vi "TimeInterpRotation2d_GetSample.vi"(9 "TimeStamp":dbl, 11 "TimeInterpRotation":T1 {"RotationValues"."SIN" format="%13.4f"; "RotationValues"."COS" format="%13.4f"; "RotationValues"."VALUE" format="%13.4f"}) -> (1 "IsPresent":bool, 3 "OutputRotation":T2={"VALUE"=0.0, "COS"=1.0, "SIN"=0.0} {"SIN" format="%13.4f"; "COS" format="%13.4f"; "VALUE" format="%13.4f"})   [LabVIEW 2019, in "Trajectory_Library.lvlib"]
doc: "Sample the buffer at the given time.\n\nInputs:\n - TimeInterpRotation2d -- Input data cluster\n - TimeStamp -- Time at which to sample (seconds)\n\nOutputs\n - OutputRotation -- Sampled Rotation2d. This is an exact value if there is a sample in the buffer at this time. Otherwise the value is interpolated. \n - IsPresent -- Returns TRUE if the buffer contains data as far back as TimeStamp."
uses:
  Trajectory_Library.lvlib
  <vilib>/gmath/NI_Gmath.lvlib
  ROTATION2D.ctl
  TypeDef/TIME_INTERPOLATABLE_ROTATION2D.ctl
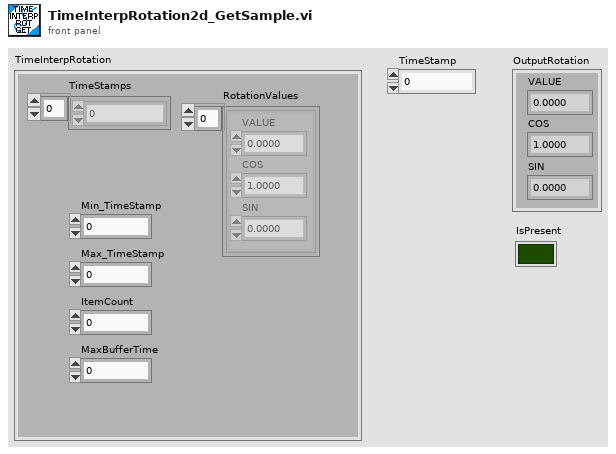
[diagram p1: front panel]
types:
  T1 = typedef "Trajectory_Library.lvlib/TIME_INTERPOLATABLE_ROTATION2D.ctl" = cluster{"TimeStamps":dbl[], "RotationValues":T2[], "Min_TimeStamp":dbl, "Max_TimeStamp":dbl, "ItemCount":i32, "MaxBufferTime":dbl}
  T2 = typedef "Trajectory_Library.lvlib/ROTATION2D.ctl" = cluster{"VALUE":dbl, "COS":dbl, "SIN":dbl}
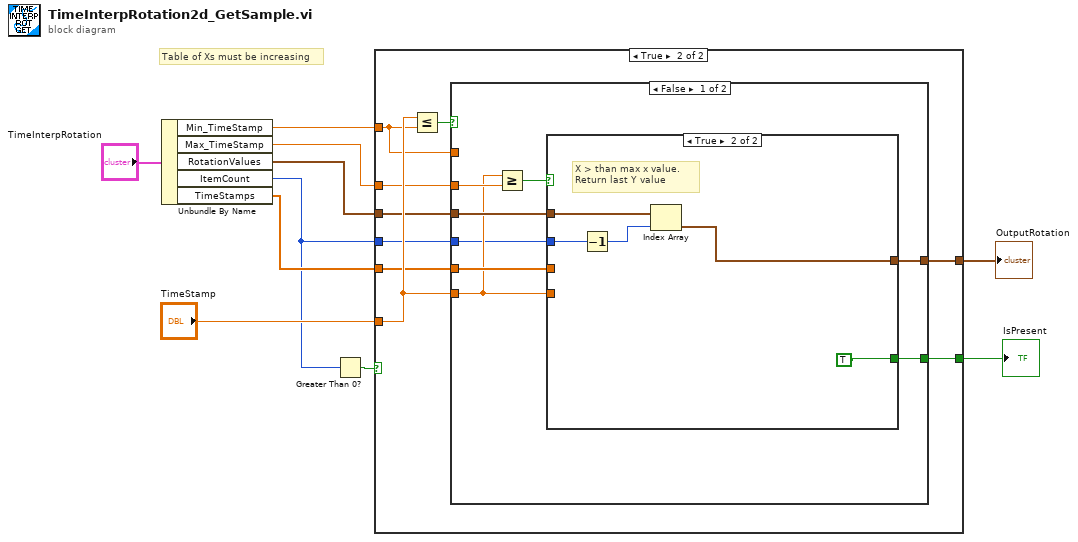
[diagram p0: block diagram]
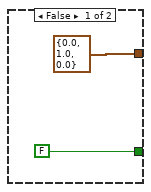
[diagram p2: hidden frame]
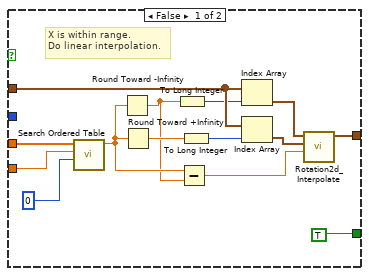
[diagram p3: hidden frame]
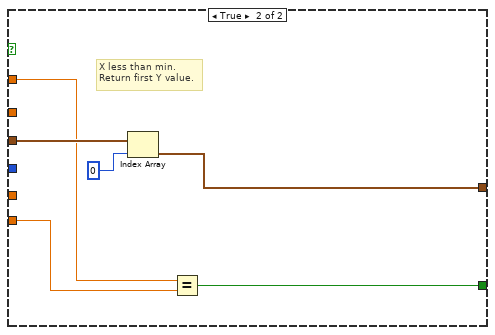
[diagram p4: hidden frame]
diagram:
  # "Table of Xs must be increasing"
  n1 = Unbundle By Name("TimeInterpRotation") -> ("Min_TimeStamp"=w7:dbl, "Max_TimeStamp"=w6:dbl, "RotationValues"=w4:T2[], "ItemCount"=w2:i32, "TimeStamps"=w5:dbl[])
  n2 = Greater Than 0?(x=w2) -> (x > 0?=w3:bool)
  n3 = case shown="True" w3 {
    tunnel: "TimeStamp" -> [_ w20]
    tunnel: [T2 {"VALUE"=0.0, "COS"=1.0, "SIN"=0.0} ("Table Y") w19] -> w9
    tunnel: w7 -> [_ w14]
    tunnel: w6 -> [_ w18]
    tunnel: w2 -> [_ w17]
    tunnel: w5 -> [_ w16]
    tunnel: w4 -> [_ w15]
    tunnel: [FALSE w13] -> w1
    frame False {
    }
    frame True {
      n4 = Less Or Equal?(x=w20, y=w14) -> (x <= y?=w21:bool)
      n5 = case shown="False" w21 {
        tunnel: w15 -> [w27 w54]
        tunnel: [w26 w52] -> w19
        tunnel: w20 -> [w24 w50]
        tunnel: w18 -> [w29 _]
        tunnel: w16 -> [w25 _]
        tunnel: w17 -> [w23 _]
        tunnel: w14 -> [_ w51]
        tunnel: [w22 w49] -> w13
        frame False {
          n6 = Greater Or Equal?(x=w24, y=w29) -> (x >= y?=w28:bool)
          n7 = case shown="True" w28 {
            tunnel: w27 -> [w39 w48]
            tunnel: [w40 w47] -> w26
            tunnel: w25 -> [w42 _]
            tunnel: w24 -> [w41 _]
            tunnel: w23 -> [_ w46]
            tunnel: [TRUE TRUE] -> w22
            frame False {
              # "X is within range.  \nDo linear interpolation."
              n8 = call <vilib>:"Search Ordered Table.vi"("starting index"=0, "x value"=w41, "ordered x array"=w42) -> ("fractional index"=w33:dbl)  [unwired: 8 in]
              n9 = Round Toward -Infinity(1:w33) -> (0:w32:dbl)
              n10 = Round Toward +Infinity(x=w33) -> (ceil(x): smallest int >= x=w34:dbl)
              n11 = To Long Integer(number=w32) -> (32bit integer=w36:i32)
              n12 = Subtract(x=w33, y=w32) -> (x-y=w31:dbl)
              n13 = To Long Integer(number=w34) -> (32bit integer=w35:i32)
              n14 = Index Array(array=w39, index=w36) -> (element=w38:T2)
              n15 = Index Array(array=w39, index=w35) -> (element=w37:T2)
              n16 = call "Rotation2d_Interpolate.vi"("T"=w31, "EncValue ROTATION"=w37, "in ROTATION"=w38) -> ("Interpolated ROTATION"=w40:T2)  [unwired: 8 in]
            }
            frame True {
              # "X > than max x value.   \nReturn last Y value"
              n17 = Decrement(x=w46) -> (x-1=w45:i32)
              n18 = Index Array(array=w48, index=w45) -> (element=w47:T2)
            }
          }
        }
        frame True {
          # "X less than min.   \nReturn first Y value."
          n19 = Index Array(array=w54, index=0) -> (element=w52:T2)
          n20 = Equal?(x=w51, y=w50) -> (x = y?=w49:bool)
        }
      }
    }
  }
  "OutputRotation" <- w9
  "IsPresent" <- w1
